vi "Intake Immediate with Deadband.vi"(0 "Left Setpoint":dbl, 1 "Right Setpoint":dbl, 2 "Deadband Value":dbl=0.01, 3 "Command Info In":T1, 4 "Description":string) -> (10 "Command Info Out":T1)   [LabVIEW 2017]
doc: "This template includes code for deadband comparision to avoid excessive command scheduling. It is particularly useful for joystick-driven commands.\n\nBe sure to right-click and select New from Template and save with a new command name."
uses:
  <vilib>/Rock Robotics/WPI/Framework/Command Status Info.ctl
  <vilib>/Rock Robotics/WPI/Framework/Completion Status.ctl
  <vilib>/Rock Robotics/WPI/Framework/Completion Notifier.ctl
  Implementation/Intake Setpoints.ctl
  Implementation/Intake Operations.ctl
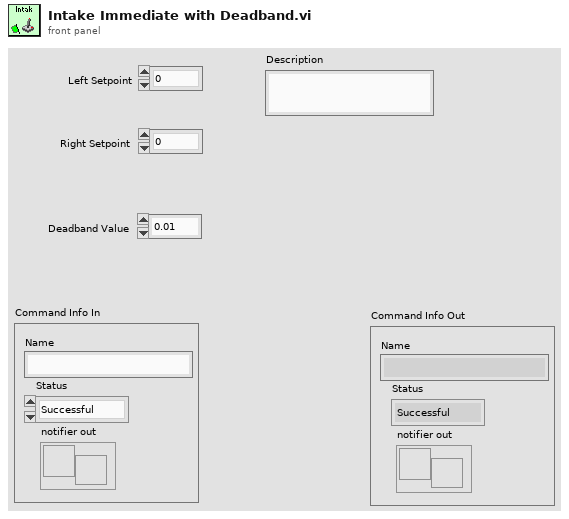
[diagram p1: front panel]
types:
  T1 = typedef "Command Status Info.ctl" = cluster{"Name":string, "Status":T2, "notifier out":T3}
  T2 = typedef "Completion Status.ctl" = enum16{"Successful", "Aborted", "Incomplete"}
  T3 = typedef "Completion Notifier.ctl" = refnum<notifier>
  T4 = typedef "Intake Setpoints.ctl" = cluster{"Operation":T5, "Left Setpoint":dbl, "Right Setpoint":dbl, "Duration":dbl}
  T5 = typedef "Intake Operations.ctl" = enum16{"Reserve", "Read Current", "Immediate", "Intake with Duration"}
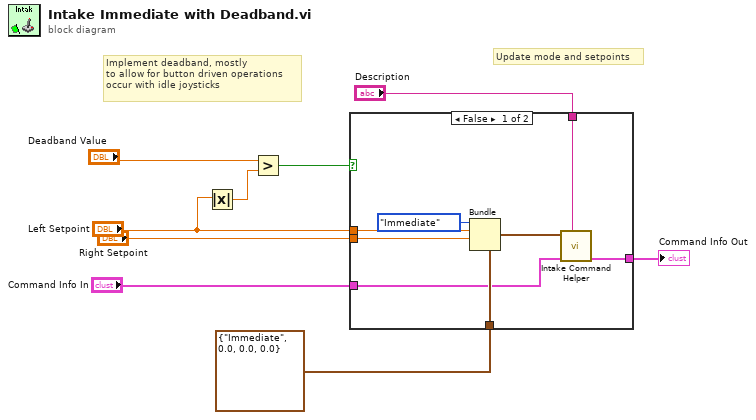
[diagram p0: block diagram]
diagram:
  # "Implement deadband, mostly\nto allow for button driven operations\noccur with idle joysticks"
  # "Update mode and setpoints"
  n1 = Absolute Value(x="Left Setpoint") -> (abs(x)=w8:dbl)
  n2 = Greater?(x="Deadband Value", y=w8) -> (0:w2:bool)
  n3 = case shown="False" w2 {
    tunnel: "Left Setpoint" -> [w12 _]
    tunnel: T4 {"Operation"=enum."Immediate", "Left Setpoint"=0.0, "Right Setpoint"=0.0, "Duration"=0.0} ("SubSystem Data") -> [w17 _]
    tunnel: [w16 w18] -> w7
    tunnel: "Command Info In" -> [w15 w18]
    tunnel: "Description" -> [w13 _]
    tunnel: "Right Setpoint" -> [w10 _]
    frame False {
      n4 = Bundle(cluster=w17, "Operation"=Intake_Operations."Immediate", "Left Setpoint"=w12, "Right Setpoint"=w10) -> (w14:T4)  [unwired: 1 in]
      n5 = call "Intake Command Helper.vi"("Description"=w13, "Command Info In"=w15, "SubSystem Data"=w14) -> ("Command Info Out"=w16:T1)  [unwired: 6 in, 2 out]
    }
    frame True {
    }
  }
  "Command Info Out" <- w7
